vi "startMaster.vi"(2 "error in (no error)":errorcluster, 3 "DAQ in":refnum<class "DAQ.lvclass">) -> (0 "error out":errorcluster, 1 "DAQ out":refnum<class "DAQ.lvclass">)   [LabVIEW 2017]
uses:
  classes/HardwareObjects/DAQ/DAQ.lvclass
  classes/HardwareObjects/DAQ/DAQ.lvclass/DAQ.ctl
  classes/HardwareObjects/DAQ/Read Master Counter Task.vi
  classes/HardwareObjects/DAQ/Write Master Counter Task.vi
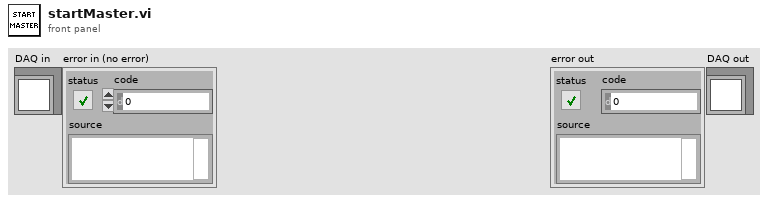
[diagram p1: front panel]
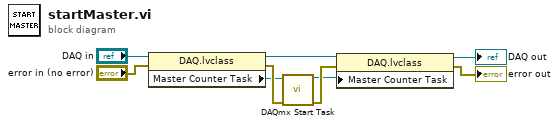
[diagram p0: block diagram]
diagram:
  n1 = property class="DAQ.lvclass"(reference="DAQ in", error in="error in (no error)") -> (reference out=w9:refnum<class "DAQ.lvclass">, error out=w6:errorcluster, "Master Counter Task"=w5:refnum<k21>)
  n2 = call <vilib>:"DAQmx Start Task.vi"("task/channels in"=w5, "error in"=w6) -> ("task out"=w7:refnum<k21>, "error out"=w8:errorcluster)  [unwired: 12 in]
  n3 = property class="DAQ.lvclass"(reference=w9, error in=w8, "Master Counter Task"=w7) -> (reference out=→"DAQ out":refnum<class "DAQ.lvclass">, error out=→"error out":errorcluster)
